vi "S7_1200 Write.vi"   [LabVIEW 2020, in "S7_1200 control.lvlib"]
uses:
  S7_1200 control.lvlib
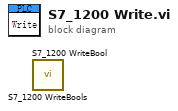
[diagram p0: block diagram]
diagram:
  n1 = call "S7_1200 WriteBools.vi"() -> ()  [unwired: 6 in, 2 out]
  n2 = call "S7_1200 WriteBool.vi"() -> ()  [unwired: 6 in, 2 out]
